vi "clump to runtime maps.vi"(4 "output dictionary":refnum<class "data dictionary.lvclass">, 6 "input dictionary":refnum<class "data dictionary.lvclass">, 7 "modbus channels":refnum<class "Modbus Module Channel.lvclass">[](array[class]), 8 "error in":errorcluster, 11 "clumps":T1[](array[typedef])) -> (0 "error out":errorcluster, 2 "output accesses":T7[](array[typedef]), 3 "input accesses":T4[](array[typedef]))   [LabVIEW 2013, in "Modbus Slave runtime.lvclass"]
uses:
  Modbus Slave runtime.lvclass
  output bulk data access.ctl
  module channel/data bank type.ctl
  data mapping elements.ctl
  <vilib>/NI/Tag Bus/tag/Data Type.ctl
  bulk data access.ctl
  module channel/Modbus Module Channel.lvclass
  <vilib>/NI/Tag Bus/dictionary/data dictionary.lvclass
  clump.ctl
  <vilib>/NI/Tag Bus Module Framework/channel/channel classification.ctl
  <vilib>/NI/Tag Bus/tag/tag descriptor.lvclass/tag descriptor.ctl
  module channel/Modbus Module Channel.lvclass/Modbus Module Channel.ctl
  <vilib>/NI/Tag Bus/tag/read data type.vi
  module channel/Read starting address.vi
  module channel/Read subindex (bool).vi
  <vilib>/NI/Tag Bus/tag/read tag name.vi
  <vilib>/NI/Tag Bus/dictionary/locate tag.vi
  <vilib>/NI/Tag Bus/tag/tag descriptor.lvclass
  <vilib>/NI/Tag Bus Module Framework/channel/TBM channel.lvclass
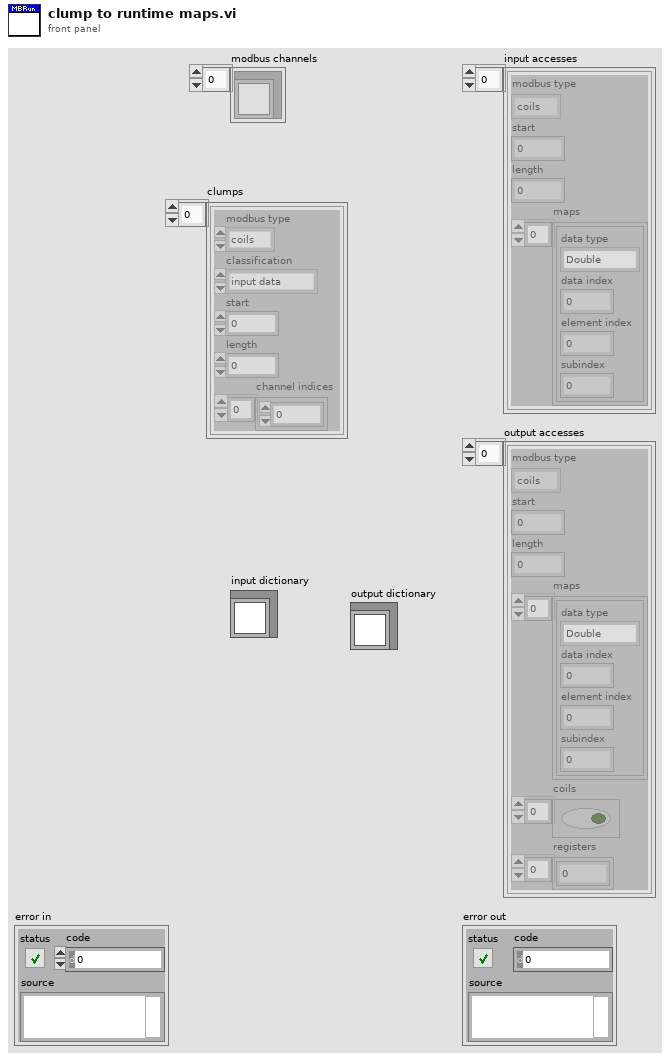
[diagram p1: front panel]
types:
  T1 = typedef "Modbus Slave runtime.lvclass/clump.ctl" = cluster{"modbus type":T2, "classification":T3, "start":i32, "length":i32, "channel indices":i32[]}
  T2 = typedef "Modbus Module Channel.lvclass/data bank type.ctl" = enum16{"coils", "discrete inputs", "input registers", "holding registers"}
  T3 = typedef "TBM channel.lvclass/channel classification.ctl" = enum16{"input data", "output data", "processing parameter", "processing result"}
  T4 = typedef "Modbus Slave runtime.lvclass/bulk data access.ctl" = cluster{"modbus type":T2, "start":u16, "length":u16, "maps":T5[]}
  T5 = typedef "Modbus Slave runtime.lvclass/data mapping elements.ctl" = cluster{"data type":T6, "data index":i32, "element index":i32, "subindex":i32}
  T6 = typedef "tag bus.lvlib/tag descriptor.lvclass/Data Type.ctl" = enum16{"Double", "Single", "I64", "I32", "I16", "I8", "U64", "U32", "U16", "U8", "Boolean", "String", "Array of Double", "Array of Single", "Array of I64", "Array of I32", "Array of I16", "Array of I8", "Array of U64", "Array of U32", "Array of U16", "Array of U8", "Array of Boolean", "Array of String"}
  T7 = typedef "Modbus Slave runtime.lvclass/output bulk data access.ctl" = cluster{"modbus type":T2, "start":u16, "length":u16, "maps":T5[], "coils":bool[], "registers":u16[]}
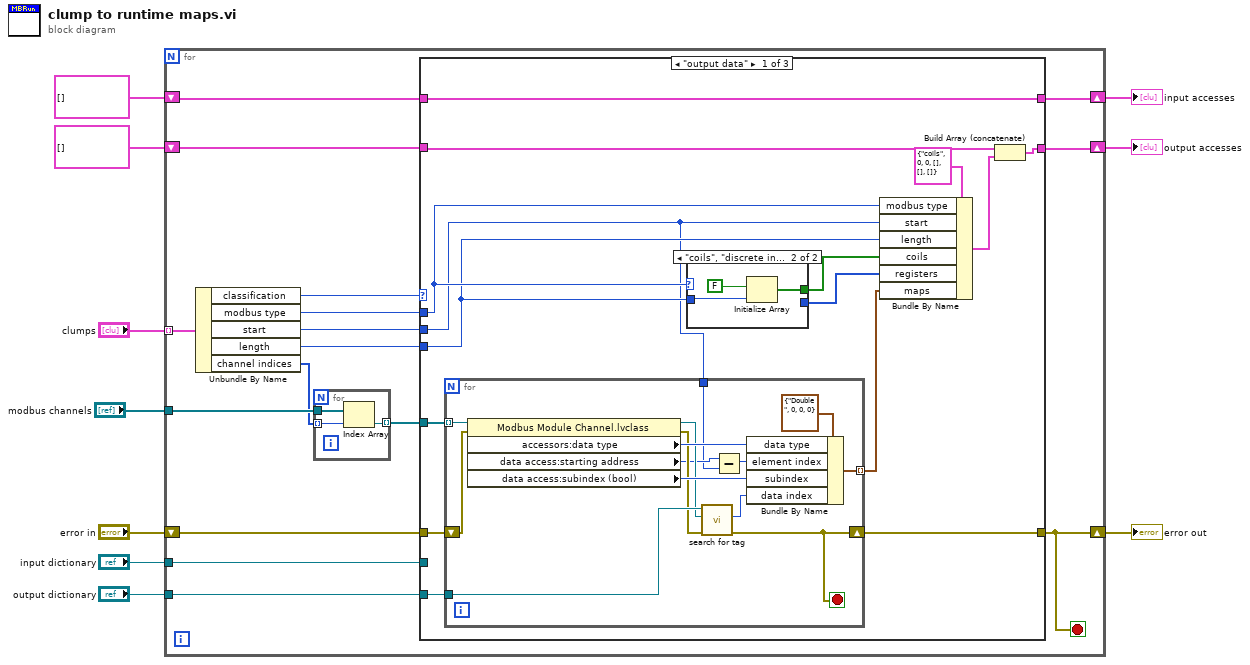
[diagram p0: block diagram]
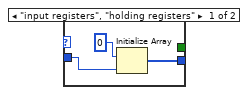
[diagram p2: hidden frame]
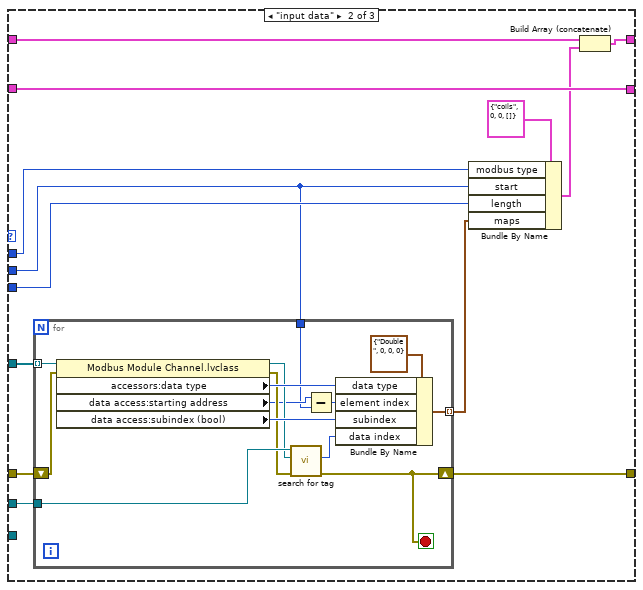
[diagram p3: hidden frame]
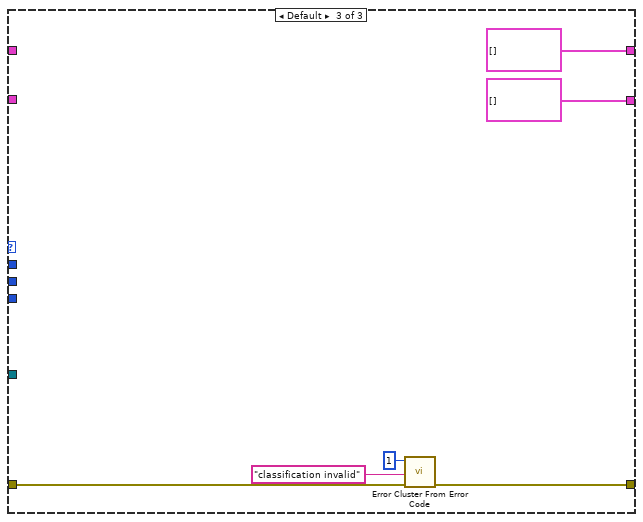
[diagram p4: hidden frame]
diagram:
  n1 = for {
    tunnel: "clumps" -> [w26] mode=indexing
    shift-right: [w20] -> w8
    shift-left: "error in" -> [w21]
    tunnel: "modbus channels" -> [w25]
    shift-right: [w22] -> w3
    shift-left: T4[] [] ("input accesses") -> [w18]
    shift-right: [w23] -> w4
    shift-left: T7[] [] ("output accesses") -> [w19]
    tunnel: "input dictionary" -> [w17]
    tunnel: "output dictionary" -> [w16]
    stop <- w20 stop-if-true
    n2 = Unbundle By Name(w26) -> ("classification"=w24:T3, "modbus type"=w15:T2, "start"=w14:i32, "length"=w13:i32, "channel indices"=w12:i32[])
    n3 = for {
      tunnel: w25 -> [w97]
      tunnel: w12 -> [w96] mode=indexing
      tunnel: [w95] -> w11 mode=indexing
      n4 = Index Array(array=w97, index=w96) -> (element=w95:refnum<class "Modbus Module Channel.lvclass">)
    }
    n5 = case shown="\"output data\"" w24 {
      tunnel: [w39 w73 T7[] [] ("output accesses")] -> w23
      tunnel: [w41 w66 T4[] [] ("input accesses")] -> w22
      tunnel: [w30 w69 w91] -> w20
      tunnel: w21 -> [w32 w70 w92]
      tunnel: w19 -> [w40 w73 _]
      tunnel: w18 -> [w41 w74 _]
      tunnel: w17 -> [_ w63 _]
      tunnel: w16 -> [w31 _ _]
      tunnel: w15 -> [w36 w72 _]
      tunnel: w14 -> [w27 w62 _]
      tunnel: w13 -> [w35 w71 _]
      tunnel: w11 -> [w28 w67 _]
      frame "output data" {
        n6 = for {
          shift-right: [w45] -> w30
          shift-left: w32 -> [w52]
          tunnel: w31 -> [w49]
          tunnel: [w54] -> w29 mode=indexing
          tunnel: w28 -> [w53] mode=indexing
          tunnel: w27 -> [w42]
          stop <- w45 stop-if-true
          n7 = property class="Modbus Module Channel.lvclass"(reference=w53, error in=w52) -> (reference out=w48:refnum<class "Modbus Module Channel.lvclass">, error out=w46:errorcluster, "accessors:data type"=w51:T6, "data access:starting address"=w43:u16, "data access:subindex (bool)"=w50:i32)
          n8 = call <vilib>:"search for tag.vi"("error in"=w46, "system tag"=w48, "data dictionary in"=w49) -> ("error out"=w45:errorcluster, "index"=w47:i32)  [unwired: 6 in, 1 out]
          n9 = Subtract(x=w43, y=w42) -> (x-y=w44:i32)
          n10 = Bundle By Name(cluster=T5 {"data type"=enum."Double", "data index"=0, "element index"=0, "subindex"=0} ("mapping element"), "data type"=w51, "element index"=w44, "subindex"=w50, "data index"=w47) -> (w54:T5)
        }
        n11 = case shown="\"coils\", \"discrete inputs\"" w36 {
          tunnel: w35 -> [w56 w61]
          tunnel: [_ w59] -> w34
          tunnel: [w58 _] -> w33
          frame "input registers", "holding registers" {
            n12 = Initialize Array(u16 0, w56) -> (w58:u16[])
          }
          frame "coils", "discrete inputs" {
            n13 = Initialize Array(FALSE, w61) -> (w59:bool[])
          }
        }
        n14 = Bundle By Name(cluster=T7 {"modbus type"=enum."coils", "start"=0, "length"=0, "maps"=[], "coils"=[], "registers"=[]} ("output data access"), "modbus type"=w36, "start"=w27, "length"=w35, "coils"=w34, "registers"=w33, "maps"=w29) -> (w37:T7)
        n15 = Build Array (concatenate)(w40, w37) -> (w39:T7[])
      }
      frame "input data" {
        n16 = for {
          shift-right: [w78] -> w69
          shift-left: w70 -> [w85]
          tunnel: w63 -> [w82]
          tunnel: [w87] -> w68 mode=indexing
          tunnel: w67 -> [w86] mode=indexing
          tunnel: w62 -> [w75]
          stop <- w78 stop-if-true
          n17 = property class="Modbus Module Channel.lvclass"(reference=w86, error in=w85) -> (reference out=w81:refnum<class "Modbus Module Channel.lvclass">, error out=w79:errorcluster, "accessors:data type"=w84:T6, "data access:starting address"=w76:u16, "data access:subindex (bool)"=w83:i32)
          n18 = call <vilib>:"search for tag.vi"("error in"=w79, "system tag"=w81, "data dictionary in"=w82) -> ("error out"=w78:errorcluster, "index"=w80:i32)  [unwired: 6 in, 1 out]
          n19 = Subtract(x=w76, y=w75) -> (x-y=w77:i32)
          n20 = Bundle By Name(cluster=T5 {"data type"=enum."Double", "data index"=0, "element index"=0, "subindex"=0} ("mapping element"), "data type"=w84, "element index"=w77, "subindex"=w83, "data index"=w80) -> (w87:T5)
        }
        n21 = Bundle By Name(cluster=T4 {"modbus type"=enum."coils", "start"=0, "length"=0, "maps"=[]} ("bulk data access"), "modbus type"=w72, "start"=w62, "length"=w71, "maps"=w68) -> (w65:T4)
        n22 = Build Array (concatenate)(w74, w65) -> (w66:T4[])
      }
      frame Default {
        n23 = call <vilib>:"Error Cluster From Error Code.vi"("error in (no error)"=w92, "error message (\"\")"="classification invalid" ("error message (\"\")"), "error code (0)"=1) -> ("error out"=w91:errorcluster)  [unwired: 6 in]
      }
    }
  }
  "output accesses" <- w4
  "input accesses" <- w3
  "error out" <- w8
